vi "Trial_1.vi"() -> ()   [LabVIEW 2019]
uses:
  <userlib>/_TI-LA/Reusable/CCS/APIs/CCS.lvlib
panel:
  out "error out":errorcluster
  out "Pass?":bool
  out "Response From Server":string
  in  "Initialize Symbol Cache?(T)":bool=TRUE
  in  "Initialize Write Cache?(T)":bool=TRUE
  in  "Run Minimized? (F)":bool
  in  "Cpus Select[]":string[](array[string])=["Any Cpu"]
  in  "Quiet Frame? (F)":bool
  in  "error in":errorcluster
  in  "CCS Base Folder":path=path "C:/ti/ccsv6/ccs_base"
  in  "CCXML File":path
  in  "Timeout (ms)":i32=60000
  in  "Port Number":u16=1444
  in  "Host Name":string="localhost"
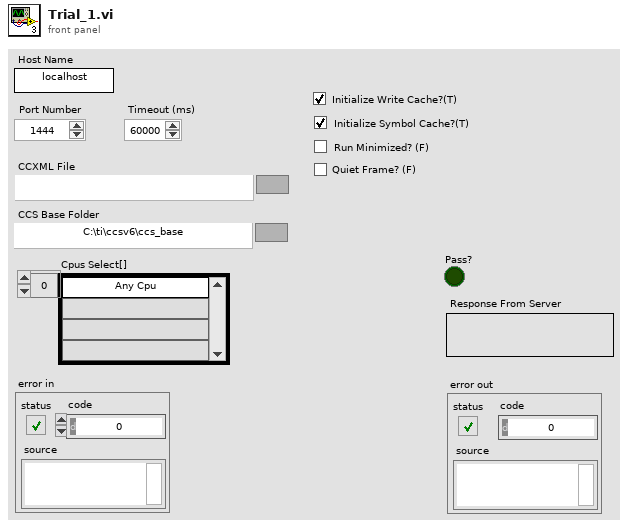
[diagram p1: front panel]
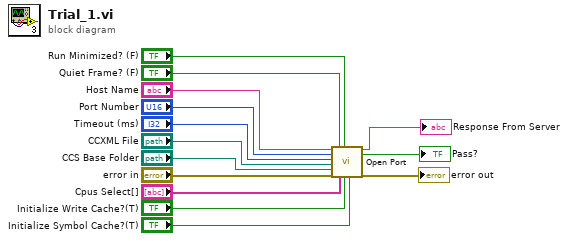
[diagram p0: block diagram]
diagram:
  n1 = call <userlib>:"Open Port.vi"("Host Name"="Host Name", "Port Number"="Port Number", "Timeout (ms)"="Timeout (ms)", "CCXML File"="CCXML File", "CCS Base Folder"="CCS Base Folder", "error in"="error in", "Quiet Frame? (F)"="Quiet Frame? (F)", "Cpus Select[]"="Cpus Select[]", "Run Minimized? (F)"="Run Minimized? (F)", "Initialize Write Cache?(T)"="Initialize Write Cache?(T)", "Initialize Symbol Cache?(T)"="Initialize Symbol Cache?(T)") -> ("Response From Server"=→"Response From Server":string, "Pass?"=→"Pass?":bool, "error out"=→"error out":errorcluster)  [unwired: 6 in]
